vi "Get Year Month Day and Seconds Values.vi"() -> (0 "seconds from 00:00":dbl format="%#.3f", 1 "day":dbl, 2 "month":dbl, 3 "year":dbl, 4 "DST?":dbl, 8 "timestamp at 00:00":timestamp, 11 "timestamp":timestamp)   [LabVIEW 2020]
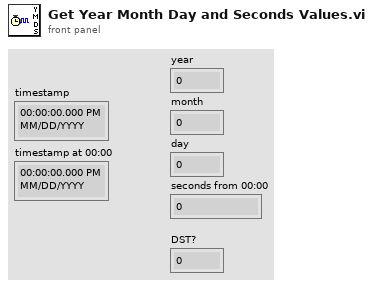
[diagram p1: front panel]
types:
  T1 = typedef "LVDateTimeRec.ctl" = cluster{"fractional second":dbl, "second":i32, "minute":i32, "hour":i32, "day of month":i32, "month":i32, "year":i32, "day of week":i32, "day of year":i32, "DST":i32}
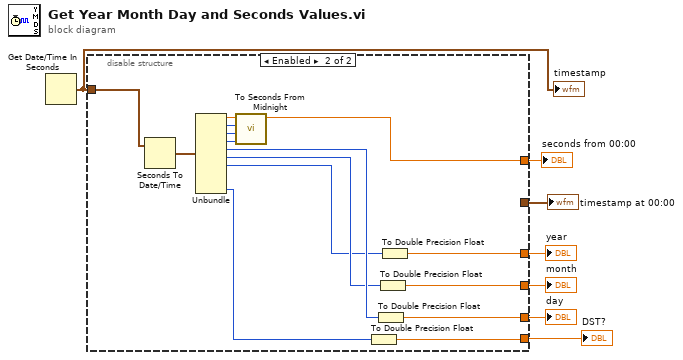
[diagram p0: block diagram]
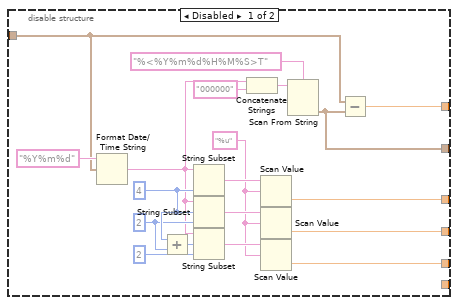
[diagram p2: hidden frame]
diagram:
  n1 = Get Date/Time In Seconds() -> (seconds since 1Jan1904=w7:timestamp)
  "timestamp" <- w7
  n2 = disable-structure shown="Enabled" {
    disable-tunnel: w7 -> [w17 w36]
    disable-tunnel: [w16 _] -> w6
    disable-tunnel: [w15 w35] -> w5
    disable-tunnel: [w10 w30] -> w4
    disable-tunnel: [w9 w29] -> w3
    disable-tunnel: [w8 w28] -> w2
    disable-tunnel: [_ w27] -> w1
    frame Disabled {
      w11 = "%u" ("format string")
      w22 = 2 ("length (rest)")
      w23 = 4 ("length (rest)")
      n3 = Format Date/Time String(time format string (%c)="%Y%m%d", seconds (now)=w17) -> (date/time string=w20:string)  [unwired: 1 in]
      n4 = Add(x=w23, y=w22) -> (x+y=w24:i32)
      n5 = String Subset(string=w20, length (rest)=w23) -> (substring=w14:string)  [unwired: 1 in]
      n6 = String Subset(string=w20, offset (0)=w23, length (rest)=w22) -> (substring=w13:string)
      n7 = String Subset(string=w20, offset (0)=w24, length (rest)=2 ("length (rest)")) -> (substring=w12:string)
      n8 = Concatenate Strings(w20, "000000" ("string")) -> (w18:string)
      n9 = Scan Value(string=w14, format string=w11) -> (value=w10:dbl)  [unwired: 1 in, 1 out]
      n10 = Scan Value(string=w13, format string=w11) -> (value=w9:dbl)  [unwired: 1 in, 1 out]
      n11 = Scan Value(string=w12, format string=w11) -> (value=w8:dbl)  [unwired: 1 in, 1 out]
      n12 = Scan From String(format string="%<%Y%m%d%H%M%S>T", input string=w18) -> (output 1=w16:timestamp)  [unwired: 3 in, 3 out]
      n13 = Subtract(x=w17, y=w16) -> (x-y=w15:dbl)
    }
    frame Enabled {
      n14 = Seconds To Date/Time(time stamp (now)=w36) -> (date time rec=w37:T1)  [unwired: 1 in]
      n15 = Unbundle(w37) -> ("fractional second"=w39:dbl, "second"=w40:i32, "minute"=w41:i32, "hour"=w38:i32, "day of month"=w34:i32, "month"=w33:i32, "year"=w32:i32, "DST"=w31:i32)  [unwired: 2 out]
      n16 = call "To Seconds From Midnight.vi"("hour"=w38, "minute"=w41, "second"=w40, "fractional second"=w39) -> ("Numeric"=w35:dbl)  [unwired: 7 in]
      n17 = To Double Precision Float(number=w31) -> (double precision float=w27:dbl)
      n18 = To Double Precision Float(number=w34) -> (double precision float=w28:dbl)
      n19 = To Double Precision Float(number=w33) -> (double precision float=w29:dbl)
      n20 = To Double Precision Float(number=w32) -> (double precision float=w30:dbl)
    }
  }
  "seconds from 00:00" <- w5
  "timestamp at 00:00" <- w6
  "year" <- w4
  "month" <- w3
  "day" <- w2
  "DST?" <- w1
